vi "Handle.vi"(7 "Queue jettl in":refnum<class "Queue jettl.lvclass">, 11 "Nominal State in":refnum<class "Nominal State.lvclass">) -> (2 "Destroy?":bool, 5 "Queue jettl out":refnum<class "Queue jettl.lvclass">)   [LabVIEW 2021, in "jettl.lvlib" / "Base Queue jettl.lvlib" / "Nominal State.lvclass"]
uses:
  Nominal State.lvclass
  Queue jettl/Queue jettl.lvclass
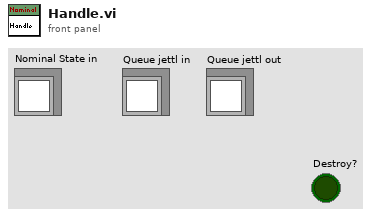
[diagram p1: front panel]
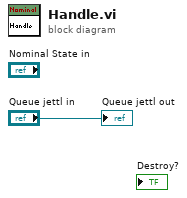
[diagram p0: block diagram]
diagram:
  "Queue jettl out" <- "Queue jettl in"
